vi "Encode.vi"(6 "Key":string, 8 "error in (no error)":errorcluster, 10 "Pretty Indent (-1=None)":i32=-1, 11 "Variant in":variant) -> (0 "error out":errorcluster, 3 "JSON out":string)   [LabVIEW 2019, in "JSON.lvlib"]
doc: "Encodes the JSON string from a LabVIEW Variant. Set <b>Pretty Indent</b> to zero to pretty print (i.e. whitespace indent) the JSON output.\n\nTo represent an empty JSON object (\"{}\") add a Cluster with an U16 Enum <b>\"empty\"</b> placeholder.\nTo represent a null JSON value (\"NULL\") add a U8 Enum <b>\"null\"</b> placholder.\nTimestamps are JSON strings formatted as defined in RFC-3339 (\"yyyy-mm-ddThh:mm:ss.uuuuuu\").\n\nCreated by: Ryan Pacini"
uses:
  JSON.lvlib
  <vilib>/Utility/Data Type/NI_Data Type.lvlib
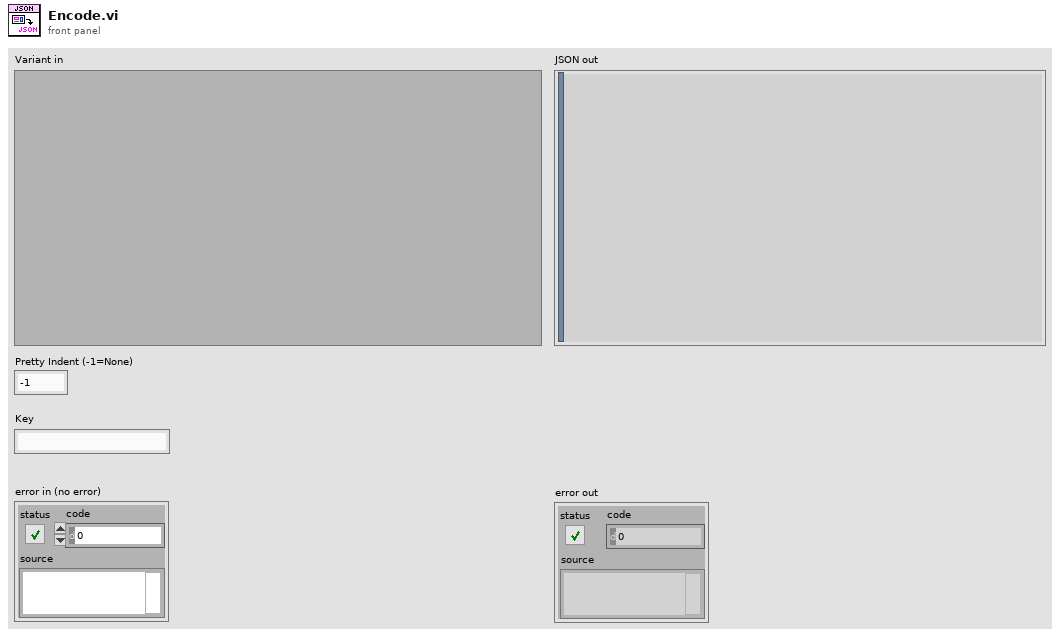
[diagram p1: front panel]
types:
  T1 = typedef "NI_Data Type.lvlib/Data Type.ctl" = enum8{"Invalid Type", "Void", "I8", "I16", "I32", "I64", "U8", "U16", "U32", "U64", "Single Float", "Double Float", "Extended Float", "Single Complex", "Double Complex", "Extended Complex", "Enum U8", "Enum U16", "Enum U32", "Enum U64", "Single Float With Unit", "Double Float With Unit", "Extended Float With Unit", "Single Complex with Unit", "Double Complex with Unit", "Extended Complex with Unit", "Boolean", "String", "Path", "Picture", "Tag", "Array", "Cluster", "Variant", "LV Variant", "Waveform", "Timestamp", "Digital Waveform", "Digital Data", "ExpressData", "Refnum", "External Data", "VI", "Poly VI", "LabVIEW Class Instance", "Fixed Point", "Set Collection", "Map Collection"}
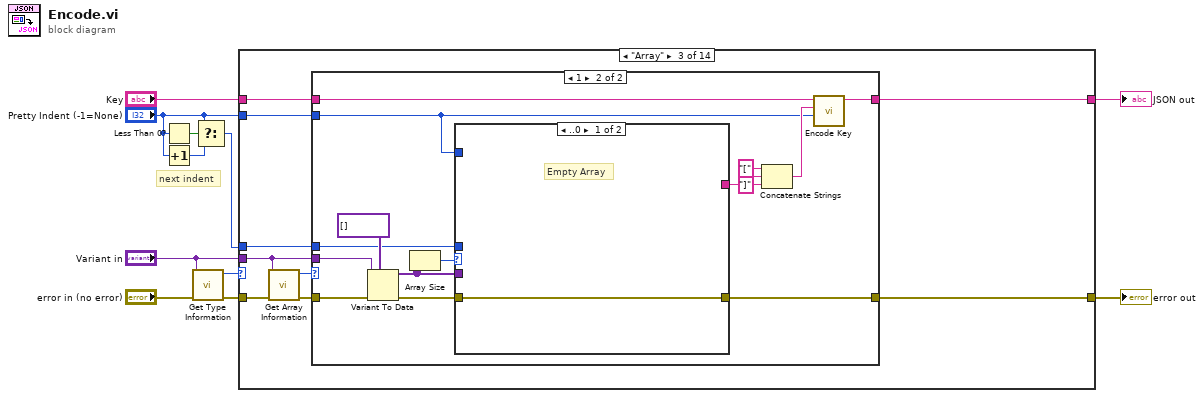
[diagram p0: block diagram]
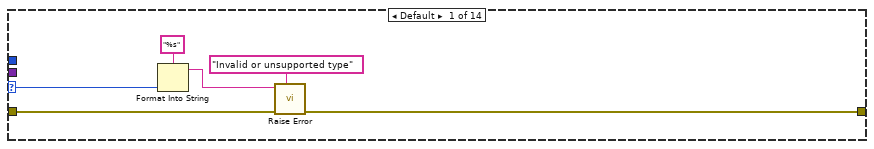
[diagram p2: hidden frame]
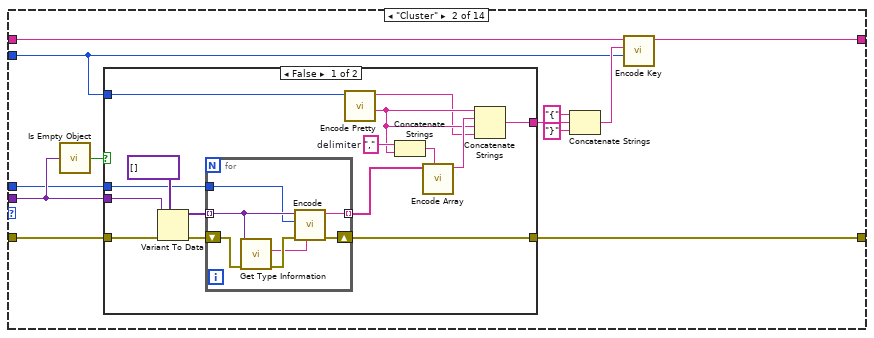
[diagram p3: hidden frame]
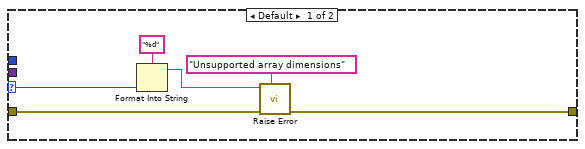
[diagram p5: hidden frame]
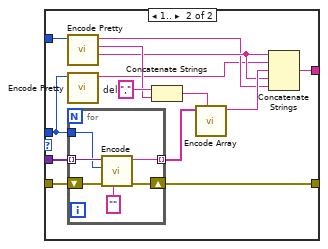
[diagram p6: hidden frame]
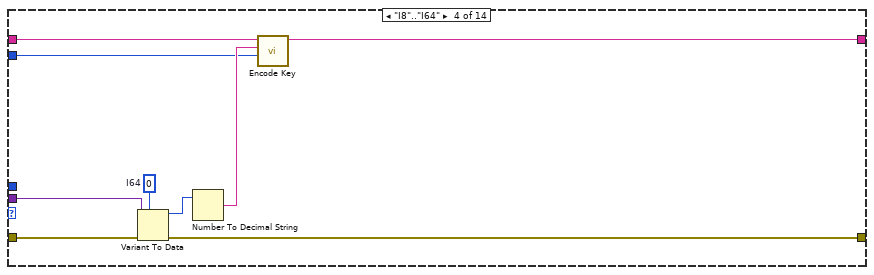
[diagram p7: hidden frame]
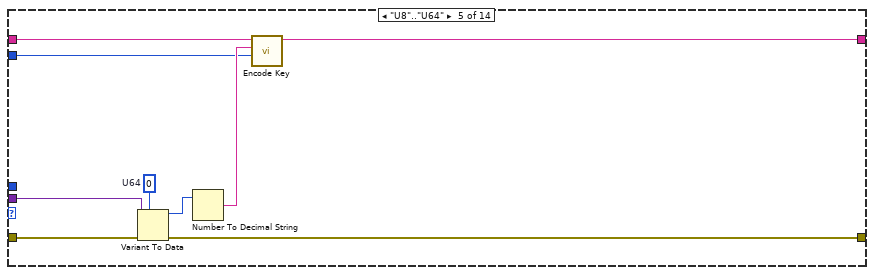
[diagram p8: hidden frame]
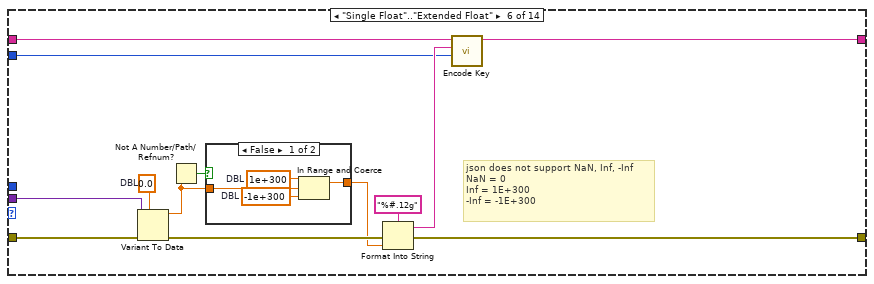
[diagram p9: hidden frame]
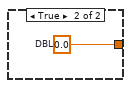
[diagram p10: hidden frame]
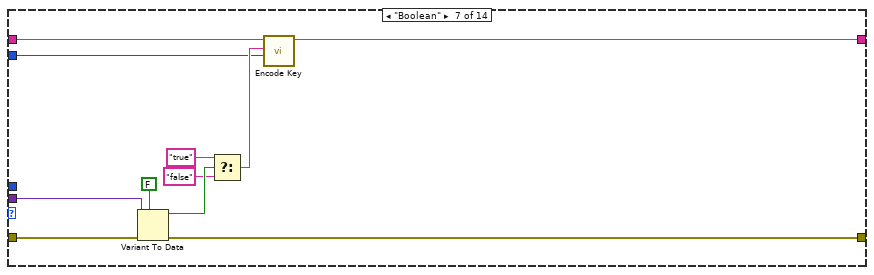
[diagram p11: hidden frame]
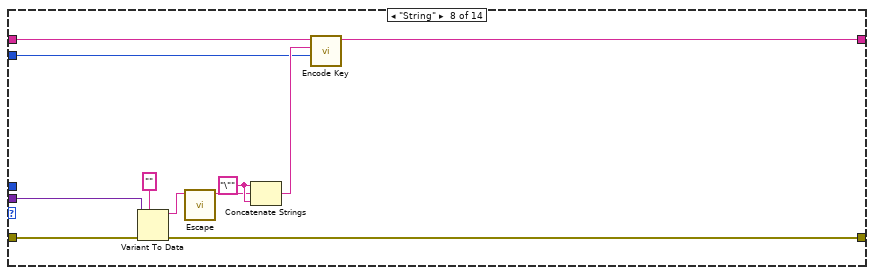
[diagram p12: hidden frame]
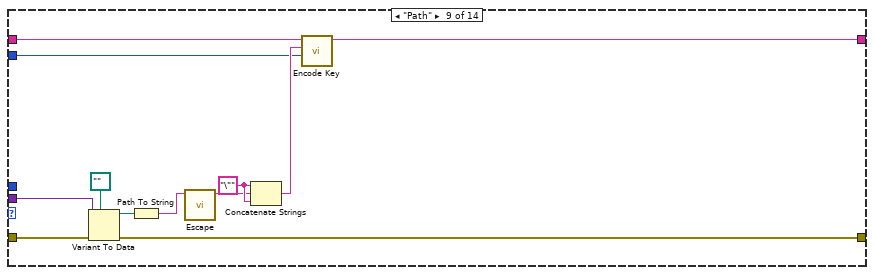
[diagram p13: hidden frame]
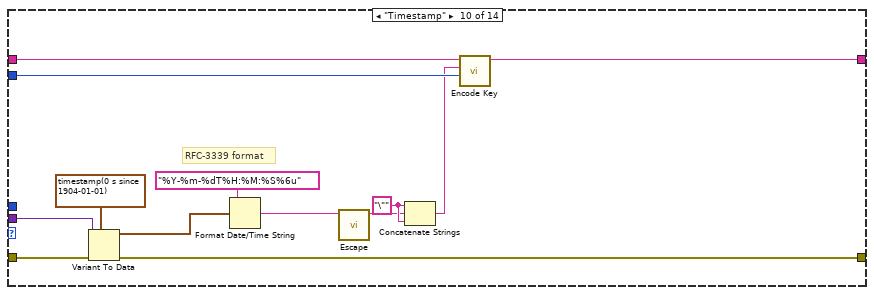
[diagram p14: hidden frame]
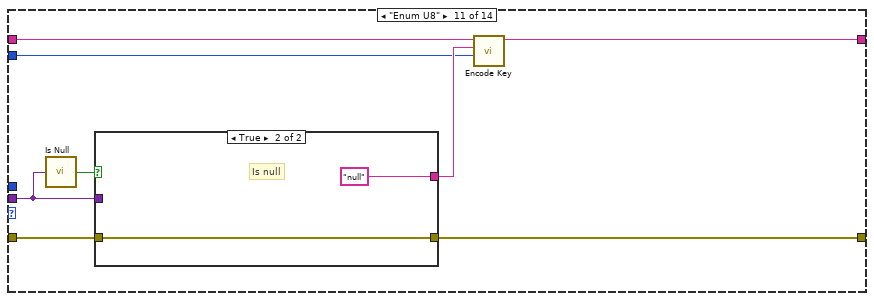
[diagram p15: hidden frame]
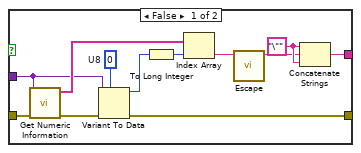
[diagram p16: hidden frame]
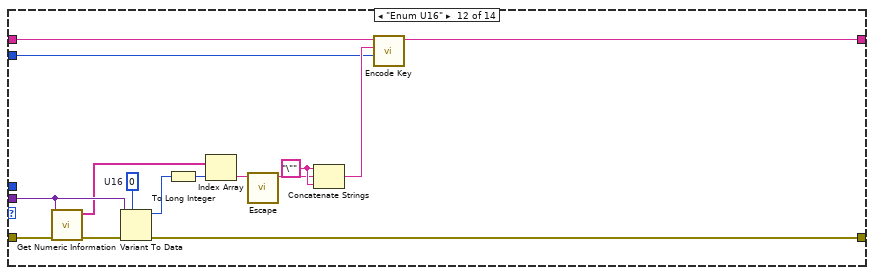
[diagram p17: hidden frame]
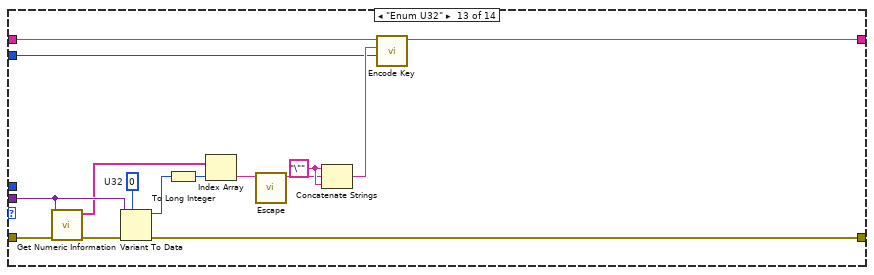
[diagram p18: hidden frame]
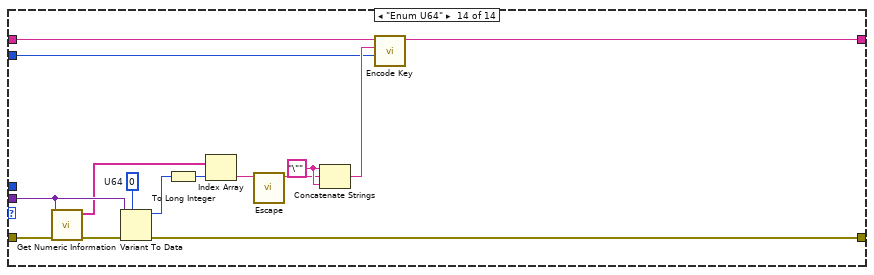
[diagram p19: hidden frame]
diagram:
  # "next indent"
  n1 = Less Than 0?(x="Pretty Indent (-1=None)") -> (x < 0?=w4:bool)
  n2 = Increment(x="Pretty Indent (-1=None)") -> (x+1=w3:i32)
  n3 = call <vilib>:"Get Type Information.vi"("error in (no error)"="error in (no error)", "variant"="Variant in") -> ("error out"=w8:errorcluster, "type"=w10:T1)  [unwired: 5 in, 3 out]
  n4 = Select(t="Pretty Indent (-1=None)", s=w4, f=w3) -> (s? t:f=w1:i32)
  n5 = case shown="\"Array\"" w10 {
    selector: w10 -> [w17 _ _ _ _ _ _ _ _ _ _ _ _ _]
    tunnel: "Variant in" -> [_ w26 w57 w111 w120 w133 w149 w160 w172 w185 w192 w219 w234 w249]
    tunnel: w8 -> [w14 w27 w58 w112 w121 w134 w150 w161 w173 w186 w193 w220 w235 w250]
    tunnel: [w13 w29 w61 w108 w117 w130 w147 w159 w171 w184 w194 w223 w238 w253] -> w7
    tunnel: [_ w24 w60 w105 w113 w125 w140 w153 w164 w174 w188 w209 w226 w240] -> w6
    tunnel: "Key" -> [_ w25 w59 w107 w116 w124 w143 w154 w165 w177 w189 w211 w227 w242]
    tunnel: w1 -> [_ w22 w54 _ _ _ _ _ _ _ _ _ _ _]
    tunnel: "Pretty Indent (-1=None)" -> [_ w18 w53 w104 w114 w122 w141 w151 w162 w176 w187 w210 w224 w239]
    frame Default {
      n6 = Format Into String(format string="%s" ("error message (\"\")"), w17) -> (resulting string=w12:string)  [unwired: 2 in, 1 out]
      n7 = call "Raise Error.vi"("message"="Invalid or unsupported type", "error in (no error)"=w14, "json"=w12) -> ("error out"=w13:errorcluster)  [unwired: 8 in]
    }
    frame "Cluster" {
      n8 = call "Is Empty Object.vi"("Value in"=w26) -> ("Is Empty Object?"=w28:bool)
      n9 = case shown="False" w28 {
        tunnel: [w44 w52] -> w29
        tunnel: w27 -> [w41 w52]
        tunnel: [w38 _] -> w23
        tunnel: w26 -> [w39 _]
        tunnel: w22 -> [w33 _]
        tunnel: w18 -> [w30 _]
        frame False {
          w35 = ","  # delimiter
          n10 = Variant To Data(error in=w41, type=variant[] [], Variant=w39) -> (data=w40:variant[], error out=w42:errorcluster)
          n11 = for {
            shift-right: [w51] -> w44
            shift-left: w42 -> [w50]
            tunnel: w40 -> [w48] mode=indexing
            tunnel: w33 -> [w46]
            tunnel: [w45] -> w37 mode=indexing
            n12 = call <vilib>:"Get Type Information.vi"("error in (no error)"=w50, "variant"=w48) -> ("error out"=w49:errorcluster, "name"=w47:string)  [unwired: 5 in, 3 out]
            n13 = call "Encode.vi"("Key"=w47, "error in (no error)"=w49, "Pretty Indent (-1=None)"=w46, "Variant in"=w48) -> ("error out"=w51:errorcluster, "JSON out"=w45:string)  [unwired: 6 in]
          }
          n14 = call "Encode Pretty.vi"("Pretty Indent (-1=None)"=w30) -> ("EOL"=w32:string, "prefix"=w31:string)  [unwired: 8 in, 1 out]
          n15 = Concatenate Strings(w35, w32) -> (w34:string)
          n16 = call "Encode Array.vi"("Delimiter (\",\")"=w34, "1D Array in"=w37) -> ("JSON out"=w36:string)  [unwired: 9 in]
          n17 = Concatenate Strings(w32, w36, w32, w31) -> (w38:string)
        }
        frame True {
          # "Is Empty Object"
        }
      }
      n18 = Concatenate Strings("{" ("string"), w23, "}" ("string")) -> (w21:string)
      n19 = call "Encode Key.vi"("Pretty Indent (-1=None)"=w18, "JSON Value"=w21, "Key (\"\"=Value only)"=w25) -> ("JSON out"=w24:string)  [unwired: 8 in]
    }
    frame "Array" {
      n20 = call <vilib>:"Get Array Information.vi"("error in (no error)"=w58, "variant"=w57) -> ("error out"=w56:errorcluster, "number of dimensions"=w55:i32)  [unwired: 6 in, 2 out]
      n21 = case shown="1" w55 {
        selector: w55 -> [w64 _]
        tunnel: [w62 w81] -> w61
        tunnel: [_ w74] -> w60
        tunnel: w59 -> [_ w75]
        tunnel: w57 -> [_ w77]
        tunnel: w56 -> [w63 w76]
        tunnel: w54 -> [_ w70]
        tunnel: w53 -> [_ w71]
        frame Default {
          n22 = Format Into String(format string="%d" ("error message (\"\")"), w64) -> (resulting string=w65:string)  [unwired: 2 in, 1 out]
          n23 = call "Raise Error.vi"("message"="Unsupported array dimensions", "error in (no error)"=w63, "json"=w65) -> ("error out"=w62:errorcluster)  [unwired: 8 in]
        }
        frame 1 {
          n24 = Variant To Data(error in=w76, type=variant[] [], Variant=w77) -> (data=w69:variant[], error out=w80:errorcluster)
          n25 = Array Size(array=w69) -> (size(s)=w68:i32)
          n26 = case shown="..0" w68 {
            tunnel: [w83 w97] -> w81
            tunnel: w80 -> [w83 w96]
            tunnel: w69 -> [_ w95]
            tunnel: [_ w92] -> w72
            tunnel: w71 -> [_ w88]
            tunnel: w70 -> [_ w85]
            frame ..0 {
              # "Empty Array"
            }
            frame 1.. {
              w91 = ","  # del
              n27 = call "Encode Pretty.vi"("Pretty Indent (-1=None)"=w88) -> ("EOL"=w87:string, "key-value gap"=w89:string, "prefix"=w86:string)  [unwired: 8 in]
              n28 = call "Encode Pretty.vi"("Pretty Indent (-1=None)"=w85) -> ("prefix"=w84:string)  [unwired: 8 in, 2 out]
              n29 = for {
                shift-right: [w103] -> w97
                shift-left: w96 -> [w101]
                tunnel: w95 -> [w102] mode=indexing
                tunnel: w85 -> [w99]
                tunnel: [w98] -> w93 mode=indexing
                n30 = call "Encode.vi"("Key"="" ("key"), "error in (no error)"=w101, "Pretty Indent (-1=None)"=w99, "Variant in"=w102) -> ("error out"=w103:errorcluster, "JSON out"=w98:string)  [unwired: 6 in]
              }
              n31 = Concatenate Strings(w91, w89) -> (w90:string)
              n32 = call "Encode Array.vi"("Delimiter (\",\")"=w90, "1D Array in"=w93) -> ("JSON out"=w94:string)  [unwired: 9 in]
              n33 = Concatenate Strings(w87, w84, w94, w87, w86) -> (w92:string)
            }
          }
          n34 = Concatenate Strings("[" ("string"), w72, "]" ("string")) -> (w73:string)
          n35 = call "Encode Key.vi"("Pretty Indent (-1=None)"=w71, "JSON Value"=w73, "Key (\"\"=Value only)"=w75) -> ("JSON out"=w74:string)  [unwired: 8 in]
        }
      }
    }
    frame "I8".."I64" {
      w110 = i64 0  # I64
      n36 = Variant To Data(error in=w112, type=w110, Variant=w111) -> (data=w109:i64, error out=w108:errorcluster)
      n37 = Number To Decimal String(number=w109) -> (decimal integer string=w106:string)  [unwired: 1 in]
      n38 = call "Encode Key.vi"("Pretty Indent (-1=None)"=w104, "JSON Value"=w106, "Key (\"\"=Value only)"=w107) -> ("JSON out"=w105:string)  [unwired: 8 in]
    }
    frame "U8".."U64" {
      w119 = u64 0  # U64
      n39 = Variant To Data(error in=w121, type=w119, Variant=w120) -> (data=w118:u64, error out=w117:errorcluster)
      n40 = Number To Decimal String(number=w118) -> (decimal integer string=w115:string)  [unwired: 1 in]
      n41 = call "Encode Key.vi"("Pretty Indent (-1=None)"=w114, "JSON Value"=w115, "Key (\"\"=Value only)"=w116) -> ("JSON out"=w113:string)  [unwired: 8 in]
    }
    frame "Single Float".."Extended Float" {
      w132 = 0.0  # DBL
      # "json does not support NaN, Inf, -Inf\nNaN = 0\nInf = 1E+300\n-Inf = -1E+300"
      n42 = Variant To Data(error in=w134, type=w132, Variant=w133) -> (data=w127:dbl, error out=w131:errorcluster)
      n43 = Not A Number/Path/Refnum?(number/path/refnum=w127) -> (NaN/Path/Refnum?=w128:bool)
      n44 = case shown="False" w128 {
        tunnel: w127 -> [w136 _]
        tunnel: [w135 w139] -> w126
        frame False {
          w137 = 1e+300  # DBL
          w138 = -1e+300  # DBL
          n45 = In Range and Coerce(upper limit=w137, x=w136, lower limit=w138) -> (coerced(x)=w135:dbl)  [unwired: 1 out]
        }
        frame True {
          w139 = 0.0  # DBL
        }
      }
      n46 = Format Into String(format string="%#.12g", error in=w131, w126) -> (resulting string=w123:string, error out=w130:errorcluster)  [unwired: 1 in]
      n47 = call "Encode Key.vi"("Pretty Indent (-1=None)"=w122, "JSON Value"=w123, "Key (\"\"=Value only)"=w124) -> ("JSON out"=w125:string)  [unwired: 8 in]
    }
    frame "Boolean" {
      n48 = Variant To Data(error in=w150, type=FALSE, Variant=w149) -> (data=w146:bool, error out=w147:errorcluster)
      n49 = Select(t="true", s=w146, f="false") -> (s? t:f=w142:string)
      n50 = call "Encode Key.vi"("Pretty Indent (-1=None)"=w141, "JSON Value"=w142, "Key (\"\"=Value only)"=w143) -> ("JSON out"=w140:string)  [unwired: 8 in]
    }
    frame "String" {
      w157 = "\"" ("string")
      n51 = Variant To Data(error in=w161, type="", Variant=w160) -> (data=w156:string, error out=w159:errorcluster)
      n52 = call "Escape.vi"("string"=w156) -> ("escaped string"=w155:string)  [unwired: 10 in]
      n53 = Concatenate Strings(w157, w155, w157) -> (w152:string)
      n54 = call "Encode Key.vi"("Pretty Indent (-1=None)"=w151, "JSON Value"=w152, "Key (\"\"=Value only)"=w154) -> ("JSON out"=w153:string)  [unwired: 8 in]
    }
    frame "Path" {
      w169 = "\"" ("string")
      n55 = Variant To Data(error in=w173, type=path "", Variant=w172) -> (data=w168:path, error out=w171:errorcluster)
      n56 = Path To String(path=w168) -> (string=w166:string)
      n57 = call "Escape.vi"("string"=w166) -> ("escaped string"=w167:string)  [unwired: 10 in]
      n58 = Concatenate Strings(w169, w167, w169) -> (w163:string)
      n59 = call "Encode Key.vi"("Pretty Indent (-1=None)"=w162, "JSON Value"=w163, "Key (\"\"=Value only)"=w165) -> ("JSON out"=w164:string)  [unwired: 8 in]
    }
    frame "Timestamp" {
      w183 = "\"" ("string")
      # "RFC-3339 format"
      n60 = Variant To Data(error in=w186, type=timestamp(0 s since 1904-01-01), Variant=w185) -> (data=w180:timestamp, error out=w184:errorcluster)
      n61 = Format Date/Time String(time format string (%c)="%Y-%m-%dT%H:%M:%S%6u", seconds (now)=w180) -> (date/time string=w178:string)  [unwired: 1 in]
      n62 = call "Escape.vi"("string"=w178) -> ("escaped string"=w182:string)  [unwired: 10 in]
      n63 = Concatenate Strings(w183, w182, w183) -> (w175:string)
      n64 = call "Encode Key.vi"("Pretty Indent (-1=None)"=w176, "JSON Value"=w175, "Key (\"\"=Value only)"=w177) -> ("JSON out"=w174:string)  [unwired: 8 in]
    }
    frame "Enum U8" {
      n65 = call "Is Null.vi"("Value in"=w192) -> ("Is Value Null?"=w191:bool)
      n66 = case shown="True" w191 {
        tunnel: [w206 w207] -> w194
        tunnel: [w205 "null"] -> w190
        tunnel: w193 -> [w202 w207]
        tunnel: w192 -> [w195 _]
        frame False {
          w197 = "\"" ("string")
          w204 = u8 0  # U8
          n67 = call <vilib>:"Get Numeric Information.vi"("error in (no error)"=w202, "variant"=w195) -> ("error out"=w203:errorcluster, "enum names"=w198:string[])  [unwired: 6 in, 2 out]
          n68 = Variant To Data(error in=w203, type=w204, Variant=w195) -> (data=w201:u8, error out=w206:errorcluster)
          n69 = To Long Integer(number=w201) -> (32bit integer=w200:i32)
          n70 = Index Array(array=w198, index=w200) -> (element=w199:string)
          n71 = call "Escape.vi"("string"=w199) -> ("escaped string"=w196:string)  [unwired: 10 in]
          n72 = Concatenate Strings(w197, w196, w197) -> (w205:string)
        }
        frame True {
          # "Is null"
        }
      }
      n73 = call "Encode Key.vi"("Pretty Indent (-1=None)"=w187, "JSON Value"=w190, "Key (\"\"=Value only)"=w189) -> ("JSON out"=w188:string)  [unwired: 8 in]
    }
    frame "Enum U16" {
      w214 = "\"" ("string")
      w222 = u16 0  # U16
      n74 = call <vilib>:"Get Numeric Information.vi"("error in (no error)"=w220, "variant"=w219) -> ("error out"=w221:errorcluster, "enum names"=w215:string[])  [unwired: 6 in, 2 out]
      n75 = Variant To Data(error in=w221, type=w222, Variant=w219) -> (data=w218:u16, error out=w223:errorcluster)
      n76 = To Long Integer(number=w218) -> (32bit integer=w217:i32)
      n77 = Index Array(array=w215, index=w217) -> (element=w216:string)
      n78 = call "Escape.vi"("string"=w216) -> ("escaped string"=w213:string)  [unwired: 10 in]
      n79 = Concatenate Strings(w214, w213, w214) -> (w212:string)
      n80 = call "Encode Key.vi"("Pretty Indent (-1=None)"=w210, "JSON Value"=w212, "Key (\"\"=Value only)"=w211) -> ("JSON out"=w209:string)  [unwired: 8 in]
    }
    frame "Enum U32" {
      w229 = "\"" ("string")
      w237 = u32 0  # U32
      n81 = call <vilib>:"Get Numeric Information.vi"("error in (no error)"=w235, "variant"=w234) -> ("error out"=w236:errorcluster, "enum names"=w230:string[])  [unwired: 6 in, 2 out]
      n82 = Variant To Data(error in=w236, type=w237, Variant=w234) -> (data=w233:u32, error out=w238:errorcluster)
      n83 = To Long Integer(number=w233) -> (32bit integer=w232:i32)
      n84 = Index Array(array=w230, index=w232) -> (element=w231:string)
      n85 = call "Escape.vi"("string"=w231) -> ("escaped string"=w228:string)  [unwired: 10 in]
      n86 = Concatenate Strings(w229, w228, w229) -> (w225:string)
      n87 = call "Encode Key.vi"("Pretty Indent (-1=None)"=w224, "JSON Value"=w225, "Key (\"\"=Value only)"=w227) -> ("JSON out"=w226:string)  [unwired: 8 in]
    }
    frame "Enum U64" {
      w244 = "\"" ("string")
      w252 = u64 0  # U64
      n88 = call <vilib>:"Get Numeric Information.vi"("error in (no error)"=w250, "variant"=w249) -> ("error out"=w251:errorcluster, "enum names"=w245:string[])  [unwired: 6 in, 2 out]
      n89 = Variant To Data(error in=w251, type=w252, Variant=w249) -> (data=w248:u64, error out=w253:errorcluster)
      n90 = To Long Integer(number=w248) -> (32bit integer=w247:i32)
      n91 = Index Array(array=w245, index=w247) -> (element=w246:string)
      n92 = call "Escape.vi"("string"=w246) -> ("escaped string"=w243:string)  [unwired: 10 in]
      n93 = Concatenate Strings(w244, w243, w244) -> (w241:string)
      n94 = call "Encode Key.vi"("Pretty Indent (-1=None)"=w239, "JSON Value"=w241, "Key (\"\"=Value only)"=w242) -> ("JSON out"=w240:string)  [unwired: 8 in]
    }
  }
  "JSON out" <- w6
  "error out" <- w7
